vi "Get Display String.vi"(11 "Int GT in":refnum<class "Int GT.lvclass">) -> (2 "Display String":string)   [LabVIEW 2018, in "Int GT.lvclass"]
uses:
  Int GT.lvclass
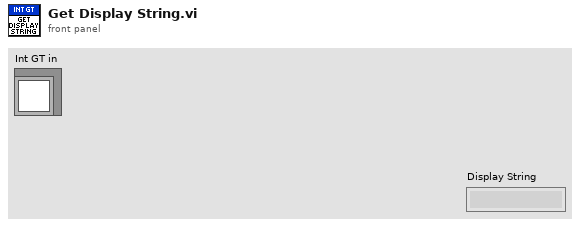
[diagram p1: front panel]
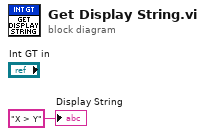
[diagram p0: block diagram]
diagram:
  "Display String" <- "X > Y" ("Display String")
